vi "relative to absolute.vi"(10 "command in":string[](array[string]), 11 "datas":T1) -> (3 "adjusted command":string[](array[string]))   [LabVIEW 2011]
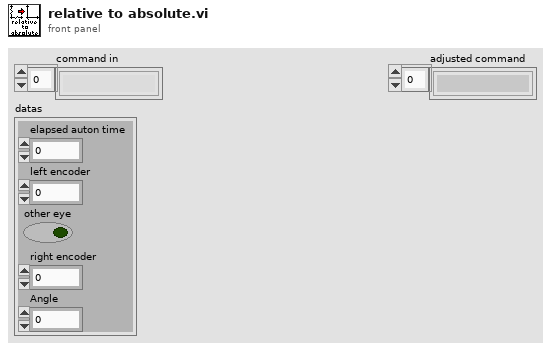
[diagram p1: front panel]
types:
  T1 = cluster{"elapsed auton time":dbl, "left encoder":dbl, "other eye":bool, "right encoder":dbl, "Angle":dbl}
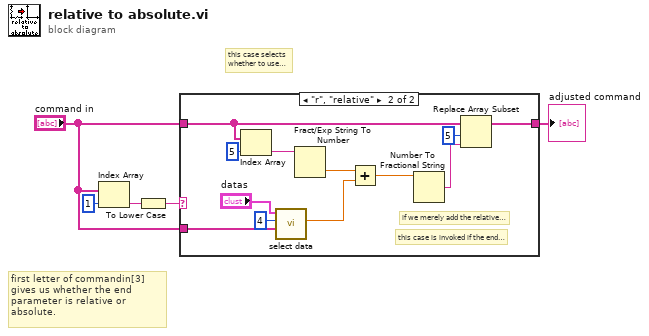
[diagram p0: block diagram]
diagram:
  # "this case selects whether to use encoders or time as the relative end parameter"
  # "first letter of commandin[3] gives us whether the end parameter is relative or absolute."
  n1 = Index Array(array="command in", index=1) -> (element=w2:string)
  n2 = To Lower Case(string=w2) -> (all lower case string=w1:string)
  n3 = case shown="\"r\", \"relative\"" w1 {
    tunnel: "command in" -> [w6 w15]
    tunnel: [w6 w14] -> w4
    tunnel: "command in" -> [_ w10]
    frame "a", "absolute", Default {
      # "absolute values.  Do nothing."
    }
    frame "r", "relative" {
      # "if we merely add the relative target value to the current value when the command is started, we get an \"absolute\" form of the relative value."
      # "this case is invoked if the end parameter is relative"
      n4 = Index Array(array=w15, index=5) -> (element=w17:string)
      n5 = call "select data.vi"("command and parameters in"=w10, "index"=u8 4, "sensor datas"="datas") -> ("accessed value"=w11:dbl)  [unwired: 8 in]
      n6 = Fract/Exp String To Number(string=w17) -> (number=w16:dbl)  [unwired: 3 in, 1 out]
      n7 = Add(x=w16, y=w11) -> (x+y=w8:dbl)
      n8 = Number To Fractional String(number=w8) -> (F-format string=w12:string)  [unwired: 3 in]
      n9 = Replace Array Subset(array=w15, new element=w12, index=5) -> (w14:string[])
    }
  }
  "adjusted command" <- w4
